vi "JAUS Observer.vi"() -> ()   [LabVIEW 2009]
uses:
  Support Files/Source ID Network Location Pair.ctl
  UDP Lib/UDP Network Location.ctl
  Support Files/Address.ctl
  Support Files/ServiceRec.ctl
  Support Files/JAUS Controller.ctl
  Support Files/Complex Services Statechart/Complex Services Queue Element.ctl
  Support Files/Complex Services Statechart/ComplexServices.lvsc/Trigger.ctl
  Support Files/VelocityState.ctl
  Support Files/TimeRec.ctl
  Support Files/LocalPose.ctl
  Support Files/NodeRec.ctl
  Support Files/ComponentRec.ctl
  <vilib>/Platform/TimedLoop/XDataNode/XDataNode.xnode
  <vilib>/Platform/TimedLoop/XDataNode/loadlvalarms.vi
  <vilib>/Platform/TimedLoop/XDataNode/timing_clust.ctl
  <vilib>/Platform/TimedLoop/XDataNode/nitl_modes.ctl
  <vilib>/Platform/TimedLoop/XDataNode/wakeup.ctl
  cRIO/Functional Global Variables/Actions for FG's.ctl
  <vilib>/Platform/TimedLoop/XDataNode/XDNodeRunTimeDep.lvlib
  Support Files/Complex Services Statechart/ComplexServices.lvsc
panel:
  out "LocalPose":T1
  out "VelocityState":T3
  out "elements":T4[](array[typedef])
  in  "Control Available?":bool=TRUE
  out "Controller out":T7={"ID"={"Subsystem Id"=90, "Node Id"=1, "Component Id"=1}, "Authority Code"=0}
  out "Init Complete out":bool
  out "Status out":u8(ring) items=["INIT", "READY", "STANDBY", "SHUTDOWN", "FAILURE", "EMERGENCY"]
  out "ServiceSeq":T8[](array[typedef])
  out "COP Info out":T9
  out "Vehicle Name out":string="Q"
  out "Vehicle ID out":T6={"Subsystem Id"=90, "Node Id"=1, "Component Id"=1}
  in  "Reset FG's":bool
  in  "stop":bool
  out "Client Records out":T10[](array[typedef])
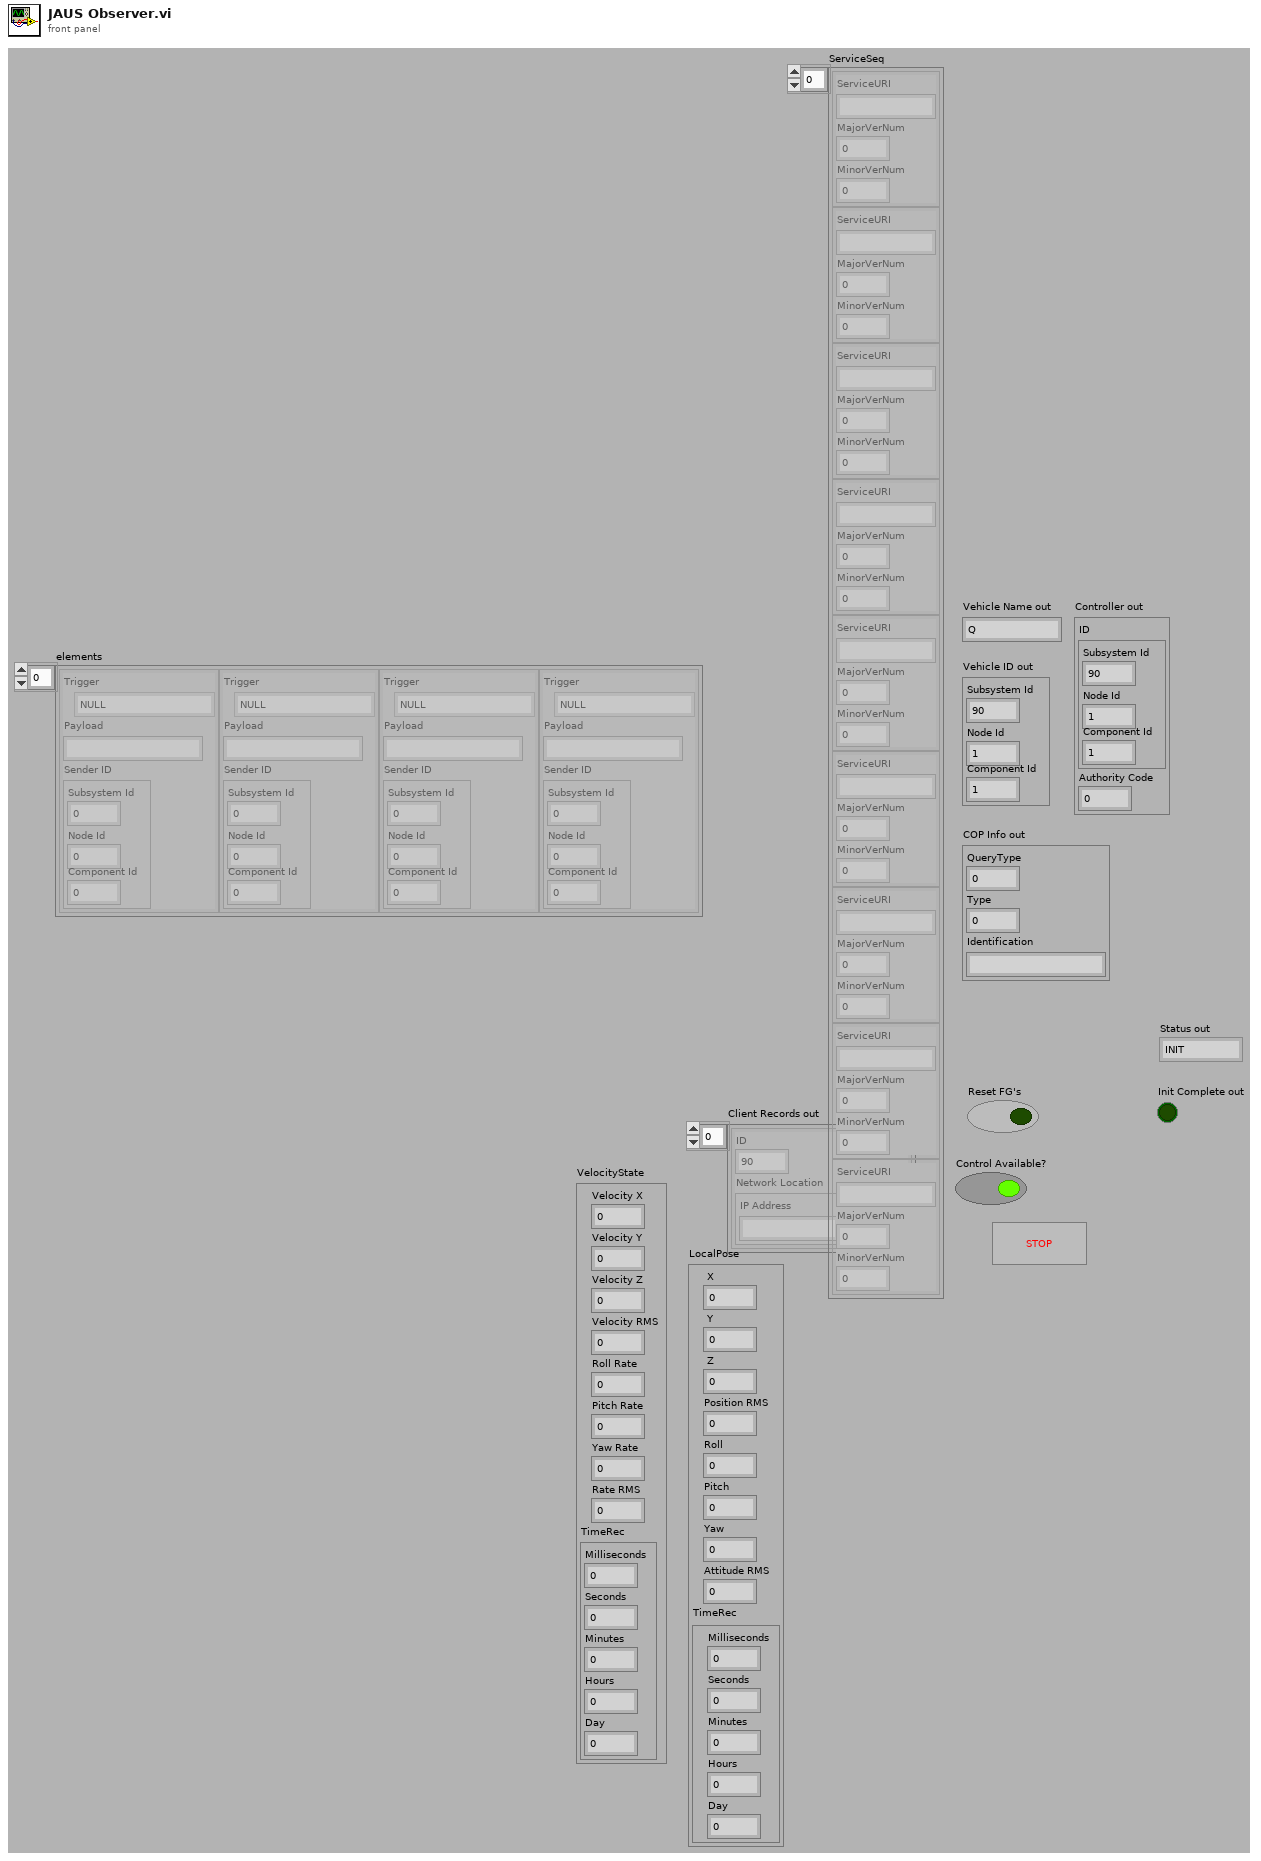
[diagram p1: front panel]
types:
  T1 = typedef "LocalPose.ctl" = cluster{" X":dbl, " Y":dbl, " Z":dbl, "Position RMS":dbl, "Roll":dbl, "Pitch":dbl, "Yaw":dbl, "Attitude RMS":dbl, "TimeRec":T2}
  T2 = typedef "TimeRec.ctl" = cluster{"Milliseconds":u32, "Seconds":u32, "Minutes":u32, "Hours":u32, "Day":u32}
  T3 = typedef "VelocityState.ctl" = cluster{"Velocity X":dbl, "Velocity Y":dbl, "Velocity Z":dbl, "Velocity RMS":dbl, "Roll Rate":dbl, "Pitch Rate":dbl, "Yaw Rate":dbl, "Rate RMS":dbl, "TimeRec":T2}
  T4 = typedef "Complex Services Queue Element.ctl" = cluster{"Trigger":T5, "Payload":string, "Sender ID":T6}
  T5 = typedef "ComplexServices.lvsc/Trigger.ctl" = enum16{"NULL", "ReceiveRequestControl", "ReceiveQueryControl", "ReceiveShutdown", "ReceiveQueryStatus", "ReceiveStandby", "ReceiveResume", "Timeout", "Initialized", "Failure", "ReceiveQueryLocalPose", "ReceiveSetLocalPose", "ReceiveQueryElementList", "ReceiveQueryElementCount", "ReceiveSetElement", "ReceiveExecuteList", "ReceiveQueryTravelSpeed", "ReceiveQueryLocalWaypoint", "ReceiveQueryActiveElement"}
  T6 = typedef "Address.ctl" = cluster{"Subsystem Id":u16, "Node Id":u8, "Component Id":u8}
  T7 = typedef "JAUS Controller.ctl" = cluster{"ID":T6, "Authority Code":u8}
  T8 = typedef "ServiceRec.ctl" = cluster{"ServiceURI":string, "MajorVerNum":u8, "MinorVerNum":u8}
  T9 = cluster{"QueryType":u8, "Type":u16, "Identification":string}
  T10 = typedef "Source ID Network Location Pair.ctl" = cluster{"ID":u32, "Network Location":T11}
  T11 = typedef "UDP Network Location.ctl" = cluster{"IP Address":string, "Port":u16}
  T12 = typedef "NodeRec.ctl" = cluster{"Node Id":u8, "ComponentSeq":T13[]}
  T13 = typedef "ComponentRec.ctl" = cluster{"Component Id":u8, "Instance Id":u8, "ServiceSeq":T8[]}
  T14 = typedef "XDNodeRunTimeDep.lvlib/timing_clust.ctl" = cluster{"Expected End [f-1]":u64, "Actual End [f-1]":u64, "Finished Late? [f-1]":bool, "Expected End [i-1]":u64, "Actual End [i-1]":u64, "Finished Late? [i-1]":bool, "Expected Start [i]":u64, "Actual Start [i]":u64, "Expected Start [f]":u64, "Actual Start [f]":u64, "Source Name":string, "Structure Name":string, "Period":i64, "Deadline":i64, "Offset":i64, "Start":i64, "Priority":i32, "Timeout":i32, "Mode":T15, "Wakeup Reason":T16, "Error":errorcluster, "Source Type":string, "Secondary Source Type":string, "Global End Time":u64, "Global Start Time":u64, "Frame Duration":u64, "Iteration Duration":u64, "Assigned CPU":i32, "I/O Scan Engine Mode":u32}
  T15 = typedef "XDNodeRunTimeDep.lvlib/nitl_modes.ctl" = enum32{"No Change", "Process missed periods, maintain original phase", "Discard missed periods, maintain original phase", "Process missed periods, ignore original phase", "Discard missed periods, ignore original phase"}
  T16 = typedef "XDNodeRunTimeDep.lvlib/wakeup.ctl" = enum32{"Normal", "Aborted", "Asynchronous wakeup", "Timing source error", "Timed loop error", "Timeout"}
  T17 = typedef "Actions for FG's.ctl" = enum16{"Read", "Write"}
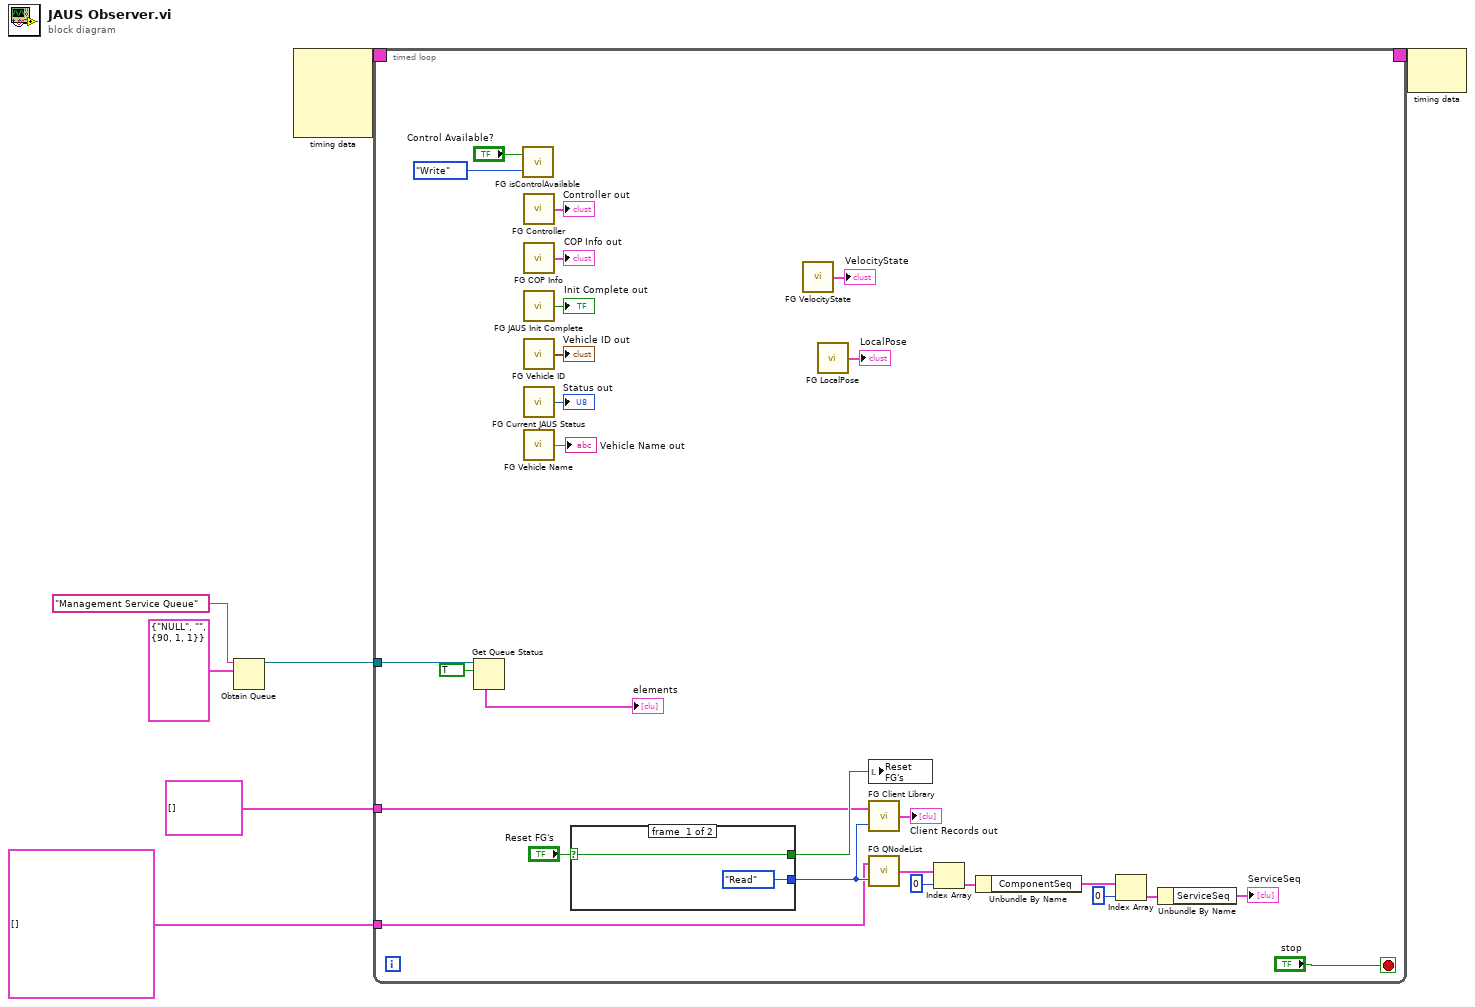
[diagram p0: block diagram]
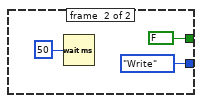
[diagram p2: hidden frame]
diagram:
  n1 = Obtain Queue(name (unnamed)="Management Service Queue", element data type=T4 {"Trigger"=enum."NULL", "Payload"="", "Sender ID"={"Subsystem Id"=90, "Node Id"=1, "Component Id"=1}} ("Receive FSM Queue Element")) -> (queue out=w1:refnum<queue>)  [unwired: 3 in, 2 out]
  n2 = node-c288() -> (w7:T14)  [unwired: 4 in]
  n3 = timed-loop {
    timing: w7 -> [_]
    timing-out: [_] -> w6
    tunnel: T12[] [] ("NodeList in") -> [w30]
    tunnel: T10[] [] ("Client Records in") -> [w29]
    tunnel: w1 -> [w12]
    stop <- "stop" stop-if-true
    n4 = Get Queue Status(queue=w12, return elements? (F)=TRUE) -> (elements=→"elements":T4[])  [unwired: 1 in, 7 out]
    n5 = call "FG isControlAvailable.vi"("FG Action (Read)"=Actions_for_FG's."Write", "isControlAvailable in"="Control Available?") -> ()  [unwired: 1 out]
    n6 = call "FG Controller.vi"() -> ("Controller out"=→"Controller out":T7)  [unwired: 2 in]
    n7 = call "FG COP Info.vi"() -> ("COP Info out"=→"COP Info out":T9)  [unwired: 2 in]
    n8 = call "FG JAUS Init Complete.vi"() -> ("Init Complete out"=→"Init Complete out":bool)  [unwired: 2 in]
    n9 = call "FG Vehicle ID.vi"() -> ("Vehicle ID out"=→"Vehicle ID out":T6)  [unwired: 2 in]
    n10 = call "FG Current JAUS Status.vi"() -> ("Status out"=→"Status out":u8)  [unwired: 2 in]
    n11 = call "FG Vehicle Name.vi"() -> ("Vehicle Name out"=→"Vehicle Name out":string)  [unwired: 2 in]
    n12 = case shown="True" "Reset FG's" {
      selector: "Reset FG's" -> [w36 _]
      tunnel: [w36 FALSE] -> w32
      tunnel: [Actions_for_FG's."Read" ("FG Action (Read)") Actions_for_FG's."Write" ("FG Action (Read)")] -> w31
      frame #0 {
      }
      frame #1 {
        n13 = Wait (ms)(milliseconds to wait=u32 50) -> ()  [unwired: 1 out]
      }
    }
    n14 = call "FG VelocityState.vi"() -> ("VelocityState out"=→"VelocityState":T3)  [unwired: 2 in]
    n15 = call "FG LocalPose.vi"() -> ("LocalPose out"=→"LocalPose":T1)  [unwired: 2 in]
    n16 = local write "Reset FG's"(w32) -> ()
    n17 = call "FG Client Library.vi"("FG Action (Read)"=w31, "Client Records in"=w29) -> ("Client Records out"=→"Client Records out":T10[])
    n18 = call "FG QNodeList.vi"("FG Action (Read)"=w31, "NodeList in"=w30) -> ("NodeList out"=w23:T12[])
    n19 = Index Array(array=w23, index=0) -> (element=w22:T12)
    n20 = Unbundle By Name(w22) -> ("ComponentSeq"=w21:T13[])
    n21 = Index Array(array=w21, index=0) -> (element=w19:T13)
    n22 = Unbundle By Name(w19) -> ("ServiceSeq"=→"ServiceSeq":T8[])
  }
  n23 = node-c288(w6) -> ()  [unwired: 1 out]
